vi "BoundaryCheck.vi"(8 "error in (no error)":errorcluster, 10 "Conf":T1, 11 "BME68x in":refnum<class "BME680.lvclass">) -> (0 "error out":errorcluster, 2 "output cluster":T1, 3 "BME68x out":refnum<class "BME680.lvclass">)   [LabVIEW 2022 SP3, in "BME680.lvlib" / "BME680.lvclass"]
uses:
  BME680.lvclass
  BME680.lvclass/BME680.ctl
  Typedefs/Conf.ctl
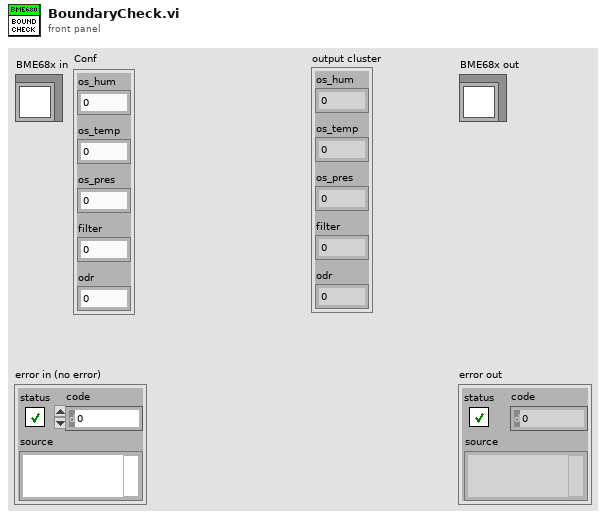
[diagram p1: front panel]
types:
  T1 = typedef "BME680.lvlib/BME680.lvclass/Conf.ctl" = cluster{"os_hum":u8, "os_temp":u8, "os_pres":u8, "filter":u8, "odr":u8}
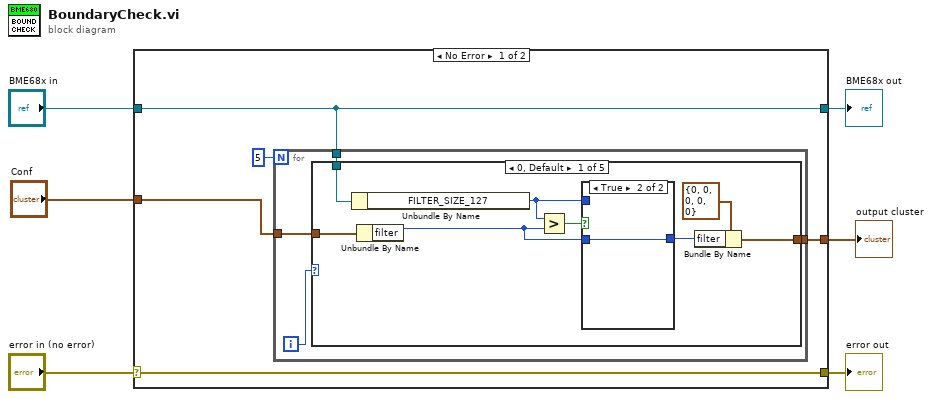
[diagram p0: block diagram]
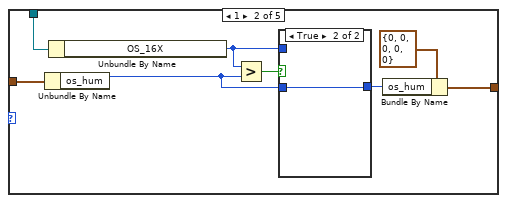
[diagram p3: hidden frame]
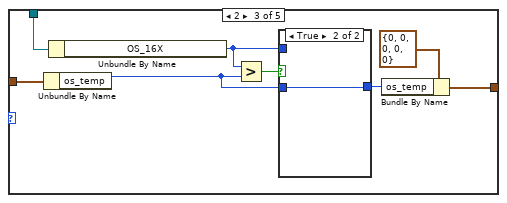
[diagram p5: hidden frame]
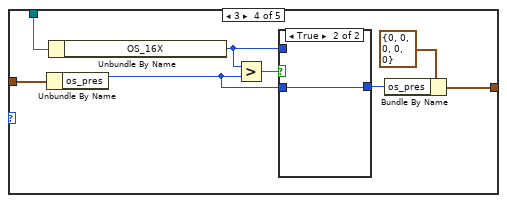
[diagram p7: hidden frame]
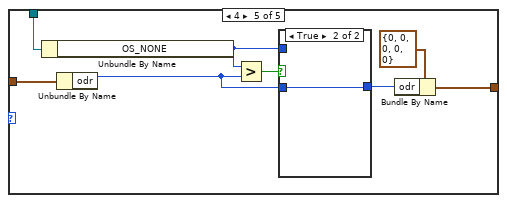
[diagram p9: hidden frame]
diagram:
  n1 = case shown="No Error" "error in (no error)" {
    selector: "error in (no error)" -> [w11 w67]
    tunnel: [w11 w67] -> w5
    tunnel: [w9 w66] -> w3
    tunnel: "BME68x in" -> [w9 w66]
    tunnel: "Conf" -> [w10 _]
    tunnel: [w8 _] -> w1
    frame No Error {
      n2 = for {
        N: 5 -> [_]
        tunnel: w10 -> [w13]
        tunnel: w9 -> [w14]
        tunnel: [w12] -> w8
        i -> [w15]
        n3 = case shown="0, Default" w15 {
          tunnel: w14 -> [w23 w33 w43 w53 w63]
          tunnel: w13 -> [w22 w32 w42 w52 w62]
          tunnel: [w16 w26 w36 w46 w56] -> w12
          frame 0, Default {
            n4 = Unbundle By Name(w23) -> ("FILTER_SIZE_127"=w19:u8)
            n5 = Unbundle By Name(w22) -> ("filter"=w20:u8)
            n6 = Greater?(x=w19, y=w20) -> (0:w21:bool)
            n7 = case shown="True" w21 {
              tunnel: [w24 w25] -> w17
              tunnel: w20 -> [_ w25]
              tunnel: w19 -> [w24 _]
              frame False {
              }
              frame True {
              }
            }
            n8 = Bundle By Name(cluster=T1 {"os_hum"=0, "os_temp"=0, "os_pres"=0, "filter"=0, "odr"=0} ("Conf"), "filter"=w17) -> (w16:T1)
          }
          frame 1 {
            n9 = Unbundle By Name(w32) -> ("os_hum"=w30:u8)
            n10 = Unbundle By Name(w33) -> ("OS_16X"=w29:u8)
            n11 = Greater?(x=w29, y=w30) -> (0:w31:bool)
            n12 = case shown="True" w31 {
              tunnel: [w34 w35] -> w27
              tunnel: w30 -> [_ w35]
              tunnel: w29 -> [w34 _]
              frame False {
              }
              frame True {
              }
            }
            n13 = Bundle By Name(cluster=T1 {"os_hum"=0, "os_temp"=0, "os_pres"=0, "filter"=0, "odr"=0} ("Conf"), "os_hum"=w27) -> (w26:T1)
          }
          frame 2 {
            n14 = Unbundle By Name(w42) -> ("os_temp"=w40:u8)
            n15 = Unbundle By Name(w43) -> ("OS_16X"=w39:u8)
            n16 = Greater?(x=w39, y=w40) -> (0:w41:bool)
            n17 = case shown="True" w41 {
              tunnel: [w44 w45] -> w37
              tunnel: w40 -> [_ w45]
              tunnel: w39 -> [w44 _]
              frame False {
              }
              frame True {
              }
            }
            n18 = Bundle By Name(cluster=T1 {"os_hum"=0, "os_temp"=0, "os_pres"=0, "filter"=0, "odr"=0} ("Conf"), "os_temp"=w37) -> (w36:T1)
          }
          frame 3 {
            n19 = Unbundle By Name(w52) -> ("os_pres"=w50:u8)
            n20 = Unbundle By Name(w53) -> ("OS_16X"=w49:u8)
            n21 = Greater?(x=w49, y=w50) -> (0:w51:bool)
            n22 = case shown="True" w51 {
              tunnel: [w54 w55] -> w47
              tunnel: w50 -> [_ w55]
              tunnel: w49 -> [w54 _]
              frame False {
              }
              frame True {
              }
            }
            n23 = Bundle By Name(cluster=T1 {"os_hum"=0, "os_temp"=0, "os_pres"=0, "filter"=0, "odr"=0} ("Conf"), "os_pres"=w47) -> (w46:T1)
          }
          frame 4 {
            n24 = Unbundle By Name(w63) -> ("OS_NONE"=w59:u8)
            n25 = Unbundle By Name(w62) -> ("odr"=w60:u8)
            n26 = Greater?(x=w59, y=w60) -> (0:w61:bool)
            n27 = case shown="True" w61 {
              tunnel: [w64 w65] -> w57
              tunnel: w60 -> [_ w65]
              tunnel: w59 -> [w64 _]
              frame False {
              }
              frame True {
              }
            }
            n28 = Bundle By Name(cluster=T1 {"os_hum"=0, "os_temp"=0, "os_pres"=0, "filter"=0, "odr"=0} ("Conf"), "odr"=w57) -> (w56:T1)
          }
        }
      }
    }
    frame Error {
    }
  }
  "error out" <- w5
  "BME68x out" <- w3
  "output cluster" <- w1
